vi "Reset.vi"(8 "error in (no error)":errorcluster, 11 "Osciloscopio in":refnum<class "Osciloscopio.lvclass">) -> (0 "error out":errorcluster, 3 "Osciloscopio out":refnum<class "Osciloscopio.lvclass">)   [LabVIEW 2020, in "Oscilloscope.lvlib" / "Osciloscopio.lvclass"]
uses:
  Osciloscopio.lvclass
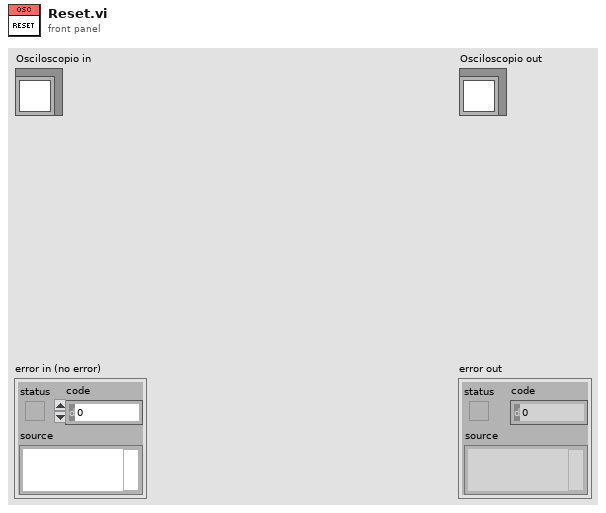
[diagram p1: front panel]
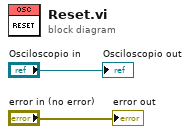
[diagram p0: block diagram]
diagram:
  "error out" <- "error in (no error)"
  "Osciloscopio out" <- "Osciloscopio in"
